vi "Add Data to History.vi"(6 "Check special fields? (F)":bool, 7 "Add to Undo?":bool, 8 "error in":errorcluster, 11 "Data in":T1={"Class"={"Ants"=refnum, "Layer"=refnum, "Templates"=refnum, "Icon"=refnum, "Glyph"=refnum, "Settings"=refnum, "Tools"=refnum}, "Ref"={"Add Layer"=refnum, "Remove Layer"=refnum, "Line Text"=[], "Body Text Spec"=refnum, "DNL_Font"=refnum, "glyph path str"=refnum, "templates path str"=refnum, "Arrow Up"=refnum, "Arrow Down"=refnum, "IE VI Ref"=refnum, "Glyphs tree"=refnum, "Templates tree"=refnum, "Layer Icon Text"=refnum, "Layer Template"=refnum, "Body Text"=refnum, "Search Templates"=refnum, "TextMarker"=refnum, "Tab Control"=refnum, "Search Glyphs"=refnum, "Line Color"=refnum, "DNL_Glyphs []"=refnum, "Fill Color"=refnum, "Tools"=refnum, "Icon"=refnum, "Preview"=refnum, "Ants"=refnum, "Terminals"=refnum, "menu reference"=refnum, "LayerNames"=[], "GlyphLoadAnimation"=refnum, "TemplateLoadAnimation"=refnum, "refreshGlyphs"=refnum, "refreshTemplates"=refnum}, "Support"={"AntsRect"={"left"=0, "top"=0, "right"=0, "bottom"=0}, "Mouse Move Coords"={"Horizontal"=0, "Vertical"=0}, "Mouse Down Coords"={"Horizontal"=0, "Vertical"=0}, "Temp Coord"={"Horizontal"=0, "Vertical"=0}, "Action"=enum."Default", "Edge Color"=4914962, "Fill Color"=16860, "Mouse Down?"=FALSE, "Draft Mode?"=FALSE, "Temp Icon"=bytes[3102], "CTRL Pressed"=FALSE, "Move Selection?"=FALSE, "AntsRect Orig"={"left"=0, "top"=0, "right"=0, "bottom"=0}, "Text"="", "TM Set?"=FALSE, "Mouse inside icon?"=FALSE, "Tool (old value)"=0, "Pencil Move Color"=0, "Swap Colors?"=FALSE, "Shift pressed?"=FALSE}}) -> (0 "error out":errorcluster, 3 "Data out":T1={"Class"={"Ants"=refnum, "Layer"=refnum, "Templates"=refnum, "Icon"=refnum, "Glyph"=refnum, "Settings"=refnum, "Tools"=refnum}, "Ref"={"Add Layer"=refnum, "Remove Layer"=refnum, "Line Text"=[], "Body Text Spec"=refnum, "DNL_Font"=refnum, "glyph path str"=refnum, "templates path str"=refnum, "Arrow Up"=refnum, "Arrow Down"=refnum, "IE VI Ref"=refnum, "Glyphs tree"=refnum, "Templates tree"=refnum, "Layer Icon Text"=refnum, "Layer Template"=refnum, "Body Text"=refnum, "Search Templates"=refnum, "TextMarker"=refnum, "Tab Control"=refnum, "Search Glyphs"=refnum, "Line Color"=refnum, "DNL_Glyphs []"=refnum, "Fill Color"=refnum, "Tools"=refnum, "Icon"=refnum, "Preview"=refnum, "Ants"=refnum, "Terminals"=refnum, "menu reference"=refnum, "LayerNames"=[], "GlyphLoadAnimation"=refnum, "TemplateLoadAnimation"=refnum, "refreshGlyphs"=refnum, "refreshTemplates"=refnum}, "Support"={"AntsRect"={"left"=0, "top"=0, "right"=0, "bottom"=0}, "Mouse Move Coords"={"Horizontal"=0, "Vertical"=0}, "Mouse Down Coords"={"Horizontal"=0, "Vertical"=0}, "Temp Coord"={"Horizontal"=0, "Vertical"=0}, "Action"=enum."Default", "Edge Color"=4914962, "Fill Color"=16860, "Mouse Down?"=FALSE, "Draft Mode?"=FALSE, "Temp Icon"=bytes[3102], "CTRL Pressed"=FALSE, "Move Selection?"=FALSE, "AntsRect Orig"={"left"=0, "top"=0, "right"=0, "bottom"=0}, "Text"="", "TM Set?"=FALSE, "Mouse inside icon?"=FALSE, "Tool (old value)"=0, "Pencil Move Color"=0, "Swap Colors?"=FALSE, "Shift pressed?"=FALSE}})   [LabVIEW 2020]
uses:
  Class/Ants/Ants.lvclass
  Class/FakedArray/FakedArray.lvclass
  vi.lib/LabVIEW Icon API/lv_icon/Classes/Icon/Icon.lvclass
  Class/Icon Library/Glyph.lvclass
  Class/Settings/Settings.lvclass
  Class/Tools/Tools Paint.lvclass
  Controls/Undo Redo Action.ctl
  <vilib>/Utility/miscctls.llb/LVPoint32TypeDef.ctl
  Controls/SupportClass_Action.ctl
  vi.lib/LabVIEW Icon API/lv_icon/Controls/IEColor.ctl
  Controls/SupportClass.ctl
  Controls/References Cluster.ctl
  vi.lib/LabVIEW Icon API/lv_icon/lv_icon.lvlib
  Controls/IE Classes.ctl
  Controls/Global Data.ctl
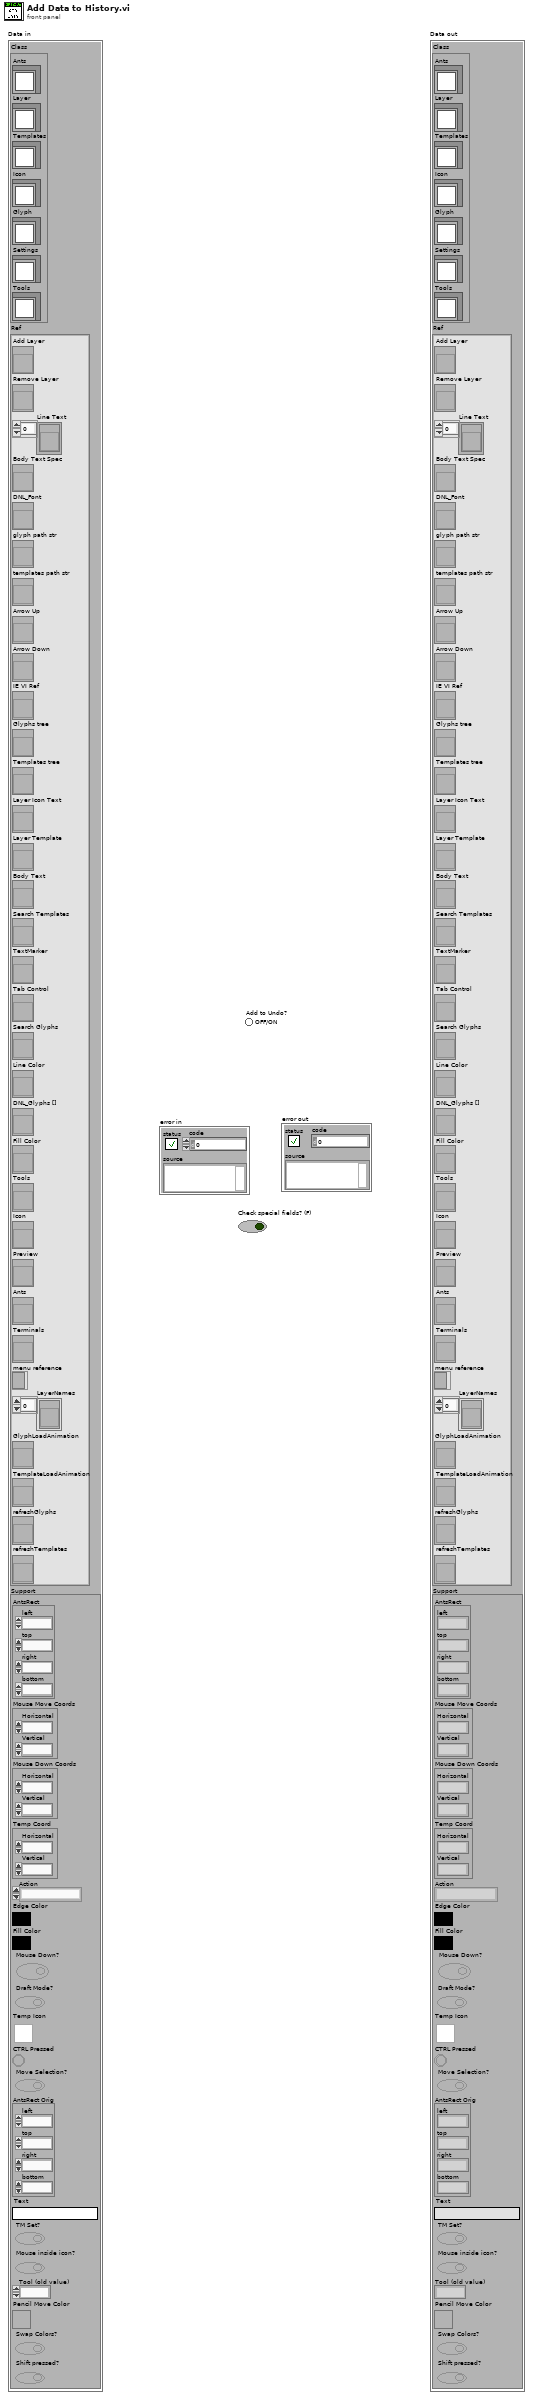
[diagram p1: front panel]
types:
  T1 = typedef "lv_icon.lvlib/Global Data.ctl" = cluster{"Class":T2, "Ref":T3, "Support":T4}
  T2 = typedef "IE Classes.ctl" = cluster{"Ants":refnum<class "Ants.lvclass">, "Layer":refnum<class "FakedArray.lvclass">, "Templates":refnum<class "FakedArray.lvclass">, "Icon":refnum<class "Icon.lvclass">, "Glyph":refnum<class "Glyph.lvclass">, "Settings":refnum<class "Settings.lvclass">, "Tools":refnum<class "Tools Paint.lvclass">}
  T3 = typedef "lv_icon.lvlib/References Cluster.ctl" = cluster{"Add Layer":refnum<vi>, "Remove Layer":refnum<vi>, "Line Text":refnum<vi>[], "Body Text Spec":refnum<vi>, "DNL_Font":refnum<vi>, "glyph path str":refnum<vi>, "templates path str":refnum<vi>, "Arrow Up":refnum<vi>, "Arrow Down":refnum<vi>, "IE VI Ref":refnum<vi>, "Glyphs tree":refnum<vi>, "Templates tree":refnum<vi>, "Layer Icon Text":refnum<vi>, "Layer Template":refnum<vi>, "Body Text":refnum<vi>, "Search Templates":refnum<vi>, "TextMarker":refnum<vi>, "Tab Control":refnum<vi>, "Search Glyphs":refnum<vi>, "Line Color":refnum<vi>, "DNL_Glyphs []":refnum<vi>, "Fill Color":refnum<vi>, "Tools":refnum<vi>, "Icon":refnum<vi>, "Preview":refnum<vi>, "Ants":refnum<vi>, "Terminals":refnum<vi>, "menu reference":refnum<k9>, "LayerNames":refnum<vi>[], "GlyphLoadAnimation":refnum<vi>, "TemplateLoadAnimation":refnum<vi>, "refreshGlyphs":refnum<vi>, "refreshTemplates":refnum<vi>}
  T4 = typedef "SupportClass.ctl" = cluster{"AntsRect":cluster{"left":i16, "top":i16, "right":i16, "bottom":i16}, "Mouse Move Coords":T5, "Mouse Down Coords":T5, "Temp Coord":T5, "Action":T6, "Edge Color":T7, "Fill Color":T7, "Mouse Down?":bool, "Draft Mode?":bool, "Temp Icon":picture, "CTRL Pressed":bool, "Move Selection?":bool, "AntsRect Orig":cluster{"left":i16, "top":i16, "right":i16, "bottom":i16}, "Text":string, "TM Set?":bool, "Mouse inside icon?":bool, "Tool (old value)":u32, "Pencil Move Color":u32, "Swap Colors?":bool, "Shift pressed?":bool}
  T5 = typedef "LVPoint32TypeDef.ctl" = cluster{"Horizontal":i32, "Vertical":i32}
  T6 = typedef "SupportClass_Action.ctl" = enum16{"Default", "Move Selection", "Glyph Library", "Tool"}
  T7 = typedef "IEColor.ctl" = u32
  T8 = typedef "Undo Redo Action.ctl" = enum16{"Init", "Add", "Undo", "Redo", "Current State"}
  T9 = cluster{"LayerIcon":picture, "LayerName":string, "Opacity":u8, "Visibility?":bool}
  T10 = typedef "Font.ctl" = string
  T11 = typedef "Alignment.ctl" = u16
  T12 = typedef "Font Size.ctl" = u8
  T13 = cluster{"Line 1 text":string, "Line 2 text":string, "Line 3 text":string, "Line 4 text":string, "Line 1 color":u32, "Line 2 color":u32, "Line 3 color":u32, "Line 4 color":u32, "Body Text Spec":cluster{"DNL_Font":T10, "Alignment":T11, "Size":T12}, "Center text vertically":bool, "Capitalize Text":bool}
  T14 = typedef "Graphic.ctl" = cluster{"Rectangle":cluster{"left":i16, "top":i16, "right":i16, "bottom":i16}, "Path":path, "Image":picture, "Filter":string, "FileName":string}
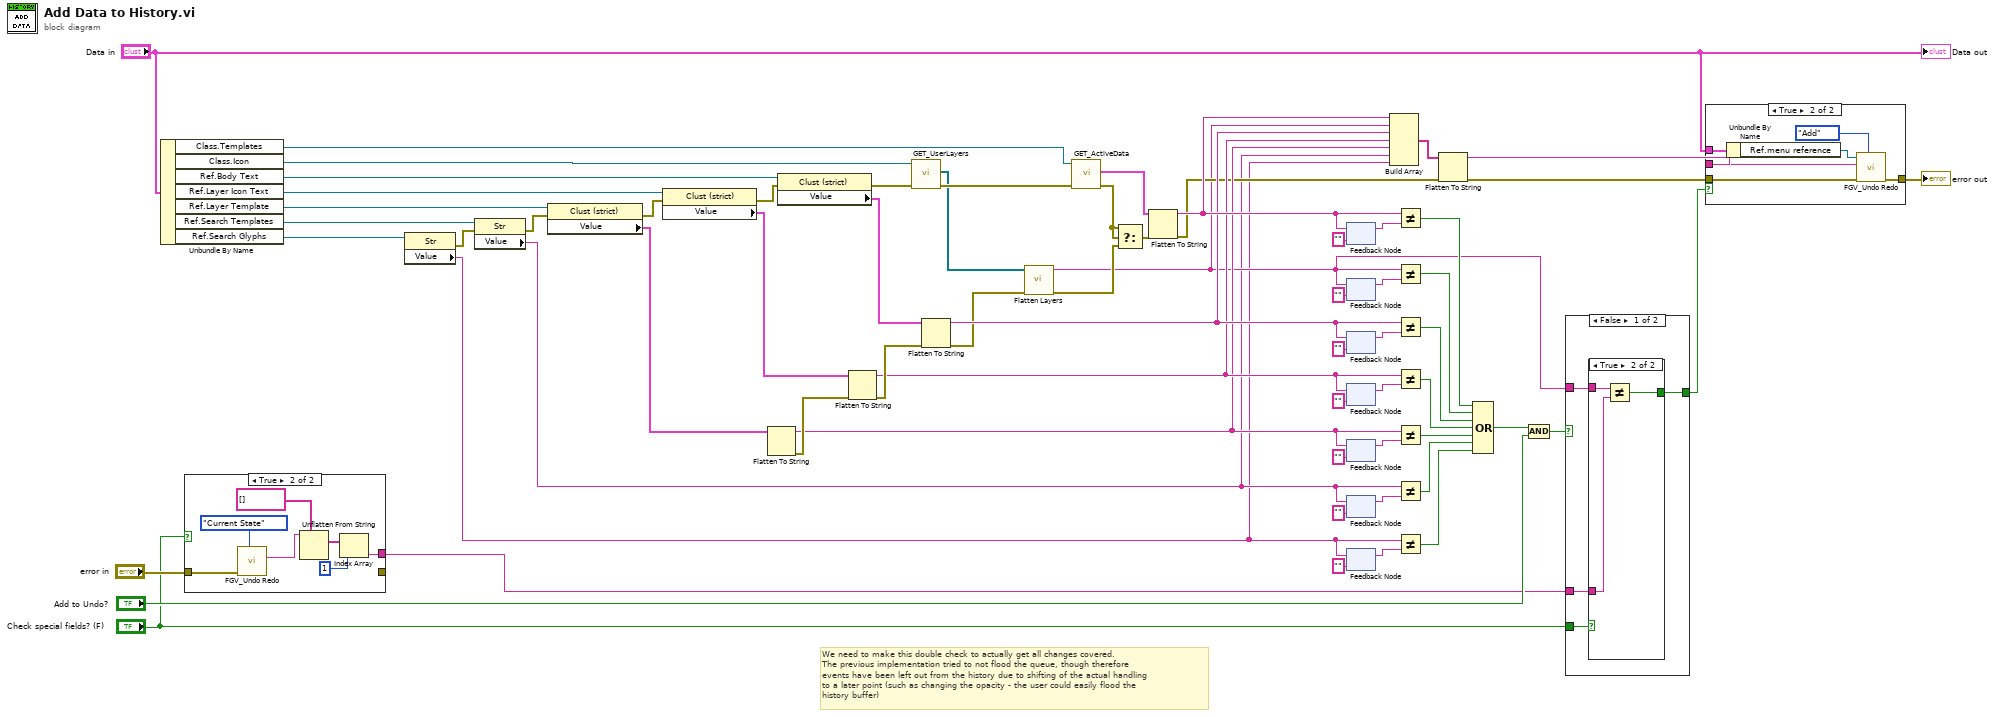
[diagram p0: block diagram]
diagram:
  # "We need to make this double check to actually get all changes covered.\nThe previous implementation tried to not flood the queue, though therefore\nevents have been left out from the history due to shifting of the actual handling\nto a later point (such as changing the opacity - the user could easily flood the\nhistory buffer)"
  n1 = Unbundle By Name("Data in") -> ("Class.Templates"=w27:refnum<class "FakedArray.lvclass">, "Class.Icon"=w29:refnum<class "Icon.lvclass">, "Ref.Body Text"=w65:refnum<vi>, "Ref.Layer Icon Text"=w64:refnum<vi>, "Ref.Layer Template"=w63:refnum<vi>, "Ref.Search Templates"=w13:refnum<vi>, "Ref.Search Glyphs"=w10:refnum<vi>)
  n2 = case shown="True" "Check special fields? (F)" {
    tunnel: "error in" -> [w66 w73]
    tunnel: [w66 _] -> _
    tunnel: [_ w68] -> w20
    frame False {
    }
    frame True {
      n3 = call "FGV_Undo Redo.vi"("Action"=Undo_Redo_Action."Current State", "error in"=w73) -> ("State Out"=w70:string)  [unwired: 4 in, 5 out]
      n4 = Unflatten From String(type=string[] [] ("appended array"), binary string=w70) -> (value=w69:string[])  [unwired: 3 in, 2 out]
      n5 = Index Array(array=w69, index=1) -> (element=w68:string)
    }
  }
  n6 = property class="Str"(reference=w10) -> (error out=w11:errorcluster, "Value"=w2:string)  [unwired: 1 in, 1 out]
  n7 = property class="Str"(reference=w13, error in=w11) -> (error out=w12:errorcluster, "Value"=w3:string)  [unwired: 1 out]
  n8 = property class="Clust (strict)"(reference=w63, error in=w12) -> (error out=w56:errorcluster, "Value"=w57:T9)  [unwired: 1 out]
  n9 = property class="Clust (strict)"(reference=w64, error in=w56) -> (error out=w51:errorcluster, "Value"=w55:T9)  [unwired: 1 out]
  n10 = Flatten To String(anything=w57) -> (data string=w33:string, error out=w50:errorcluster)  [unwired: 1 in, 3 out]
  n11 = property class="Clust (strict)"(reference=w65, error in=w51) -> (error out=w28:errorcluster, "Value"=w52:T13)  [unwired: 1 out]
  n12 = Flatten To String(anything=w55, error in (no error)=w50) -> (data string=w34:string, error out=w49:errorcluster)  [unwired: 3 out]
  n13 = call-dynamic "GET_UserLayers.vi"("error in (no error)"=w28, "Icon.lvclass in"=w29) -> ("error out"=w26:errorcluster, "All Layers"=w14:refnum<class "Layer.lvclass">[])  [unwired: 8 out]
  n14 = Flatten To String(anything=w52, error in (no error)=w49) -> (data string=w35:string, error out=w17:errorcluster)  [unwired: 3 out]
  n15 = call "Flatten Layers.vi"("Error In"=w17, "Layers"=w14) -> ("Error Out"=w16:errorcluster, "String"=w15:string)  [unwired: 8 in]
  n16 = call-dynamic "GET_ActiveData.vi"("error in (no error)"=w26, "FakedArray in"=w27) -> ("error out"=w38:errorcluster, "Path & Icon"=w44:T14)  [unwired: 8 out]
  n17 = Select(t=w38, s=w38, f=w16) -> (s? t:f=w37:errorcluster)
  n18 = Flatten To String(anything=w44, error in (no error)=w37) -> (data string=w36:string, error out=w30:errorcluster)  [unwired: 3 out]
  n19 = feedback-in #1(w36) -> ()
  n20 = feedback #1("" ("data string")) -> (w46:string)
  n21 = feedback-in #2(w15) -> ()
  n22 = feedback #2("" ("data string")) -> (w47:string)
  n23 = feedback-in #3(w35) -> ()
  n24 = feedback #3("" ("data string")) -> (w54:string)
  n25 = feedback-in #4(w34) -> ()
  n26 = feedback #4("" ("data string")) -> (w58:string)
  n27 = feedback-in #5(w33) -> ()
  n28 = feedback #5("" ("data string")) -> (w61:string)
  n29 = feedback #6("" ("data string")) -> (w8:string)
  n30 = feedback-in #6(w3) -> ()
  n31 = feedback #7("" ("data string")) -> (w7:string)
  n32 = feedback-in #7(w2) -> ()
  n33 = Build Array(w36, w15, w35, w34, w33, w3, w2) -> (w32:string[])
  n34 = Not Equal?(x=w36, y=w46) -> (x != y?=w39:bool)
  n35 = Not Equal?(x=w15, y=w47) -> (x != y?=w40:bool)
  n36 = Not Equal?(x=w35, y=w54) -> (x != y?=w41:bool)
  n37 = Not Equal?(x=w34, y=w58) -> (x != y?=w42:bool)
  n38 = Not Equal?(x=w33, y=w61) -> (x != y?=w43:bool)
  n39 = Not Equal?(x=w3, y=w8) -> (x != y?=w5:bool)
  n40 = Not Equal?(x=w2, y=w7) -> (x != y?=w4:bool)
  n41 = Flatten To String(anything=w32, error in (no error)=w30) -> (data string=w22:string, error out=w31:errorcluster)  [unwired: 3 out]
  n42 = Compound Arithmetic op=OR(w39, w40, w41, w42, w43, w5, w4) -> (w24:bool)
  n43 = And(x=w24, y="Add to Undo?") -> (x .and. y?=w19:bool)
  n44 = case shown="False" w19 {
    selector: w19 -> [_ w81]
    tunnel: [w75 w81] -> w23
    tunnel: w15 -> [w77 _]
    tunnel: w20 -> [w76 _]
    tunnel: "Check special fields? (F)" -> [w74 _]
    frame False {
      n45 = case shown="True" w74 {
        tunnel: w77 -> [_ w80]
        tunnel: w76 -> [_ w79]
        tunnel: [_ w78] -> w75
        frame False {
        }
        frame True {
          n46 = Not Equal?(x=w80, y=w79) -> (x != y?=w78:bool)
        }
      }
    }
    frame True {
    }
  }
  n47 = case shown="True" w23 {
    tunnel: [w82 w87] -> w62
    tunnel: w31 -> [w82 w86]
    tunnel: w22 -> [_ w85]
    tunnel: "Data in" -> [_ w84]
    frame False {
    }
    frame True {
      n48 = Unbundle By Name(w84) -> ("Ref.menu reference"=w83:refnum<k9>)
      n49 = call "FGV_Undo Redo.vi"("Action"=Undo_Redo_Action."Add", "error in"=w86, "State In"=w85, "menu reference"=w83) -> ("error out"=w87:errorcluster)  [unwired: 2 in, 5 out]
    }
  }
  "error out" <- w62
  "Data out" <- "Data in"
